vi "Automatic CE-CERT Inverter MODBUS TCP-IP Curtailment and Power Factor (Reduced Time)v2(multiple inverters).vi"() -> ()   [LabVIEW 2018]
uses:
  7c97fb1c-71e2-46b6-83e0-b90824be2fa8.vi
  af948a96-4452-4f5d-91ce-aeaf404a94af.vi
  83a0a89a-57e4-4031-9348-eb6639a1bf24.vi
  f3cab8c3-2d05-4b9a-baf3-8a451c362fa6.vi
  3941be6d-a080-493a-893c-1af352c84378.vi
  1a821f27-6730-4aaa-ab64-43c28f9c5f35.vi
  749368e9-8a13-4457-ac74-086f0bb157c2.vi
  1ca09a49-d2c4-4d2a-8422-a7731fce5b7b.vi
  a7e399ce-82dc-48aa-a6e2-ac362b8dfa23.vi
  75f83434-2c83-437c-aa7d-48cbf84b3d36.vi
  6cf8bfcf-bab5-4fe0-9dd9-fe191ab04daa.vi
  010fc5d1-faf8-4fdd-ade0-65e49e8fa1d8.vi
  614cc60f-aada-4277-8735-aed6e9796954.vi
  2032eeee-5097-44a1-b1ee-3eaf9e39defa.vi
  4bf1f800-a3f2-4091-8e61-355c803042a3.vi
  9cb70969-7b0c-4217-9893-0bce95bddca2.vi
  a7de19d3-9b8c-4fa7-88a3-467bd0df0b9d.vi
  8c202147-daa6-4192-8d63-29ec7b4b5446.vi
  <vilib>/Plasmionique/MB Master/MB_Master_TCP/MB_Master_TCP.lvclass
  C:/Program Files (x86)/National Instruments/LabVIEW 2018/vi.lib/Plasmionique/MB Master/MB_Master/MB_Master.lvclass
  <vilib>/Plasmionique/MB Master/MB Master.lvlib
panel:
  in  "1086 Inverter IP":string
  in  "1200 Inverter IP":string
  in  "Inverter Select":T1(ring)
  out "Setup Complete":bool
  in  "1084 Inverter IP":string
  out "Setup Runtime (s)":u32
  in  "Setup Curtailment and Power Factor":bool
  out "Curtailment Complete":bool
  out "Power Factor Complete":bool
  out "Power Factor Runtime (s)":u32
  out "Curtailment Runtime (s)":u32
  in  "Stop Button":bool
  in  "Send Power Factor":bool
  in  "Send Curtailment":bool
  in  "Curtailment % (28-100)":u16
  in  "Power Factor Setpoint":i32
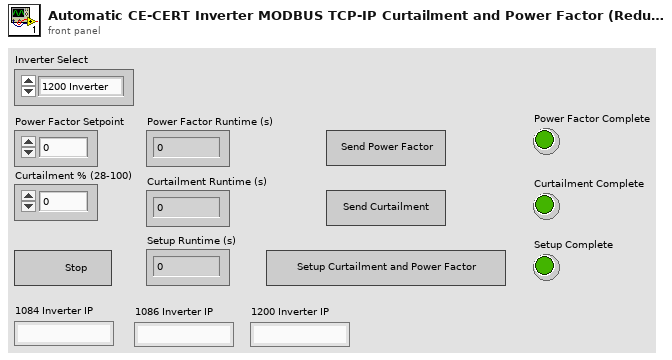
[diagram p1: front panel]
types:
  T1 = enum16{"1200 Inverter", "1084 Inverter", "1086 Inverter"}
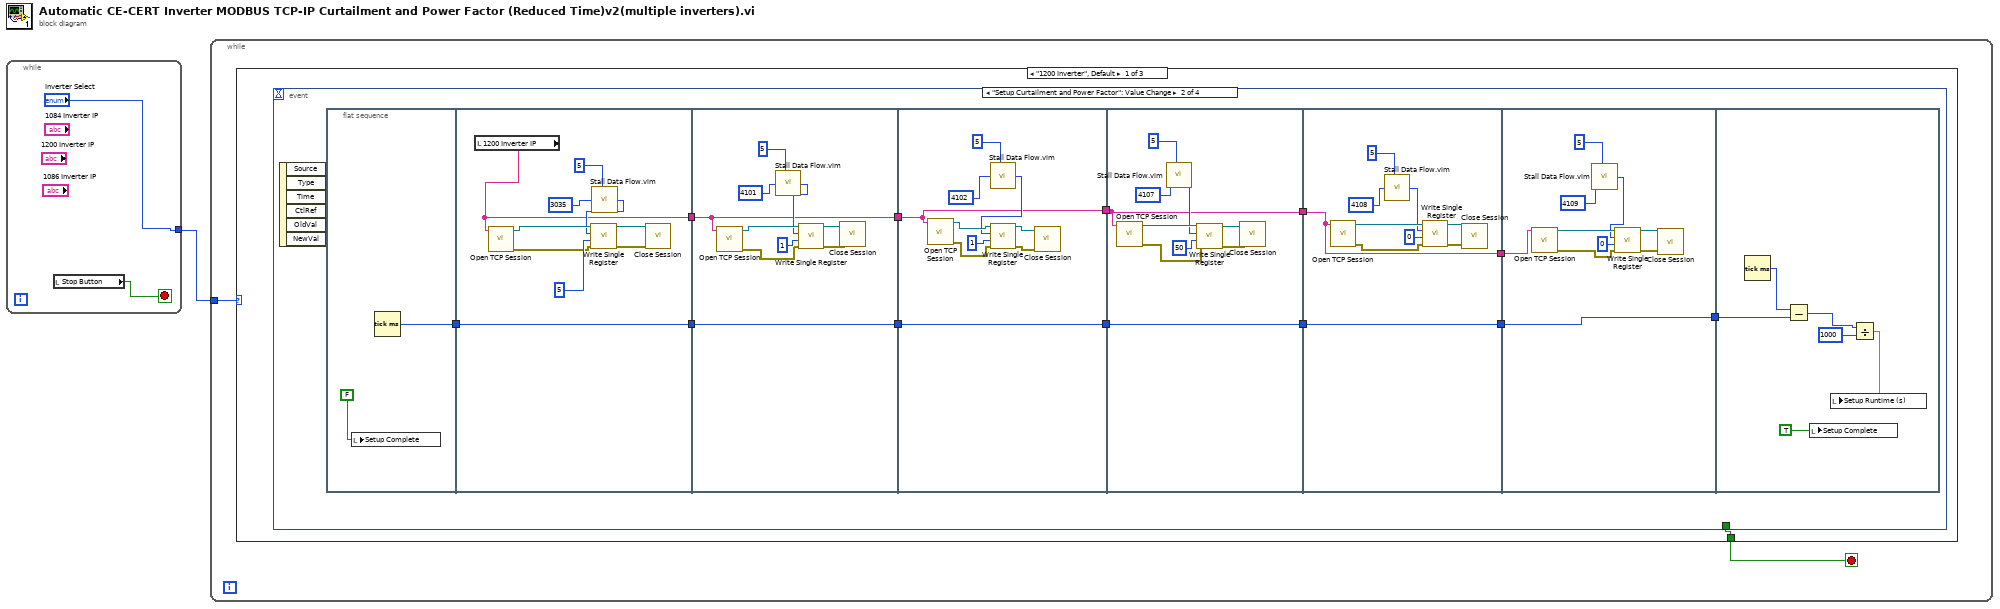
[diagram p0: block diagram]
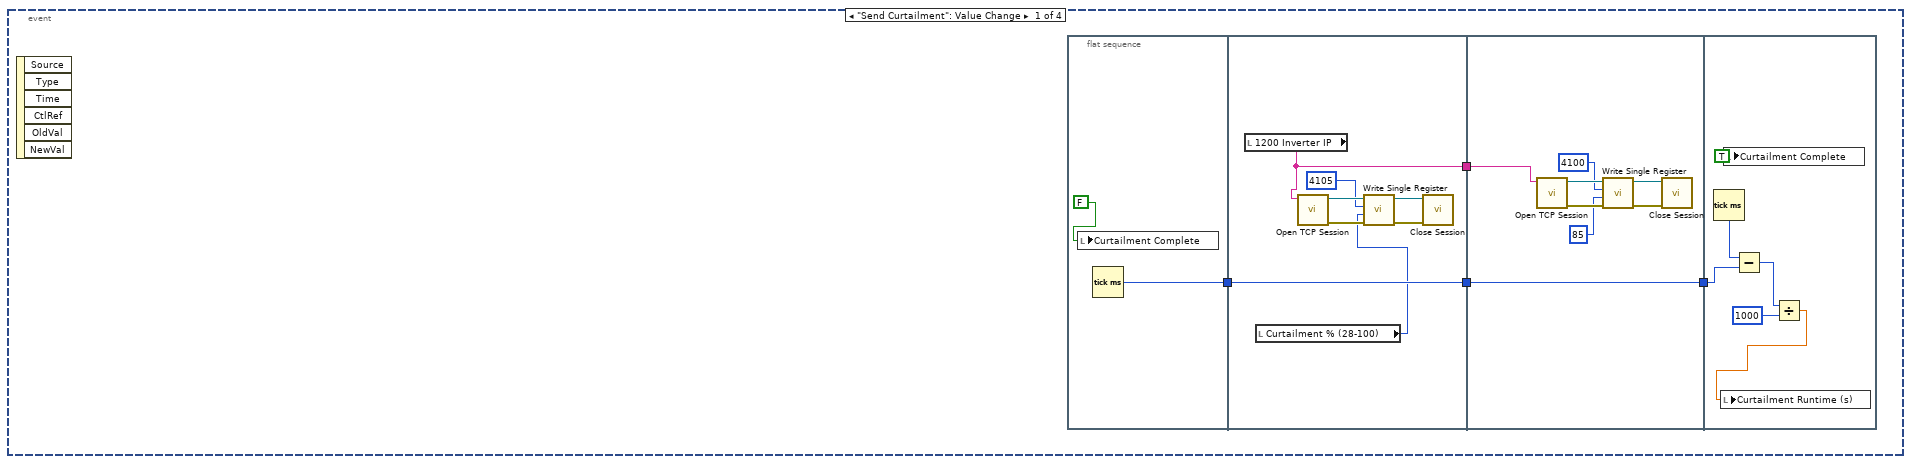
[diagram p2: hidden frame]
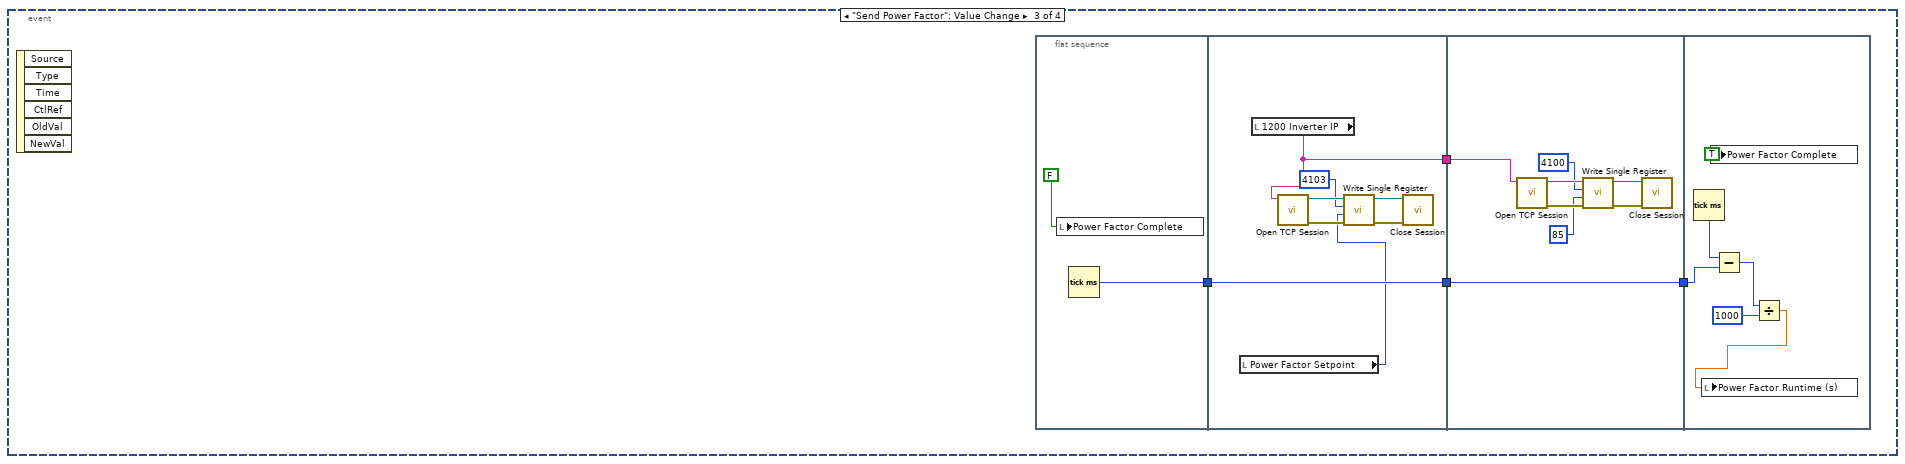
[diagram p3: hidden frame]
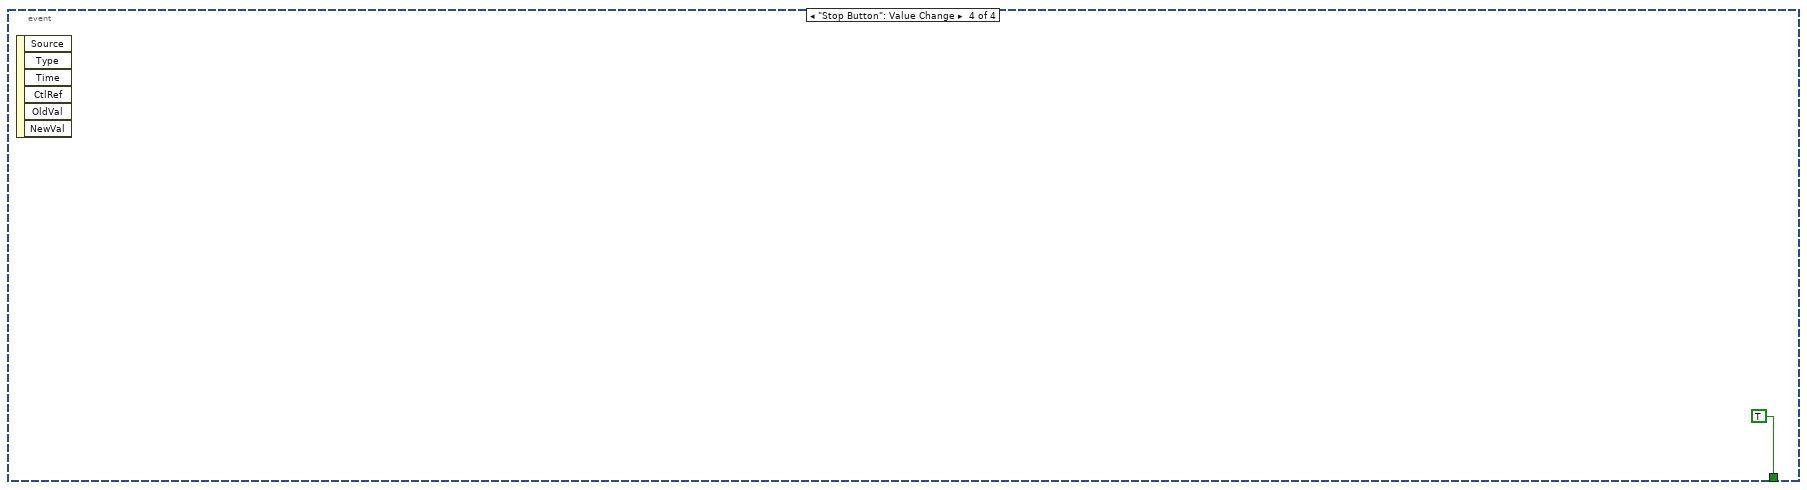
[diagram p4: hidden frame]
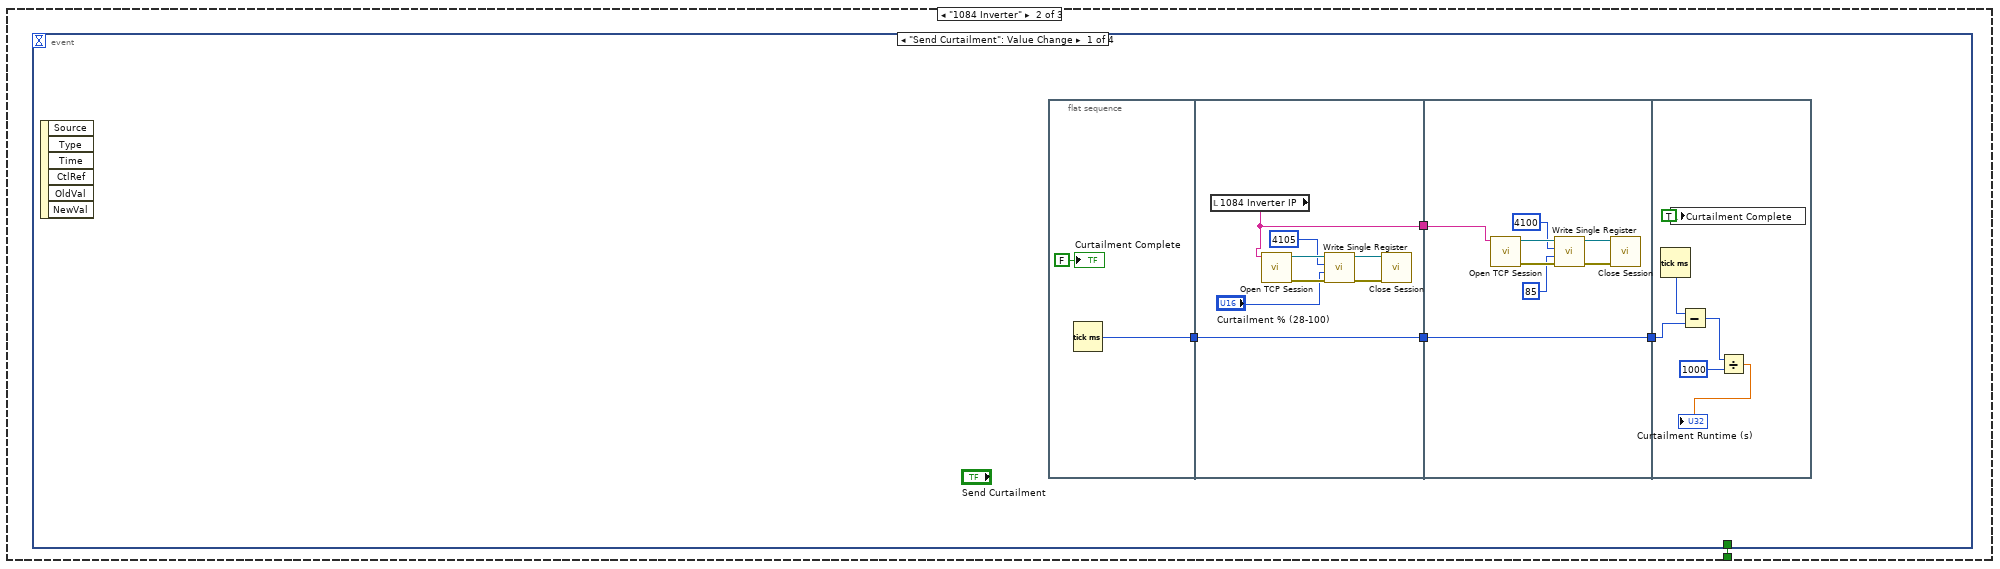
[diagram p5: hidden frame]
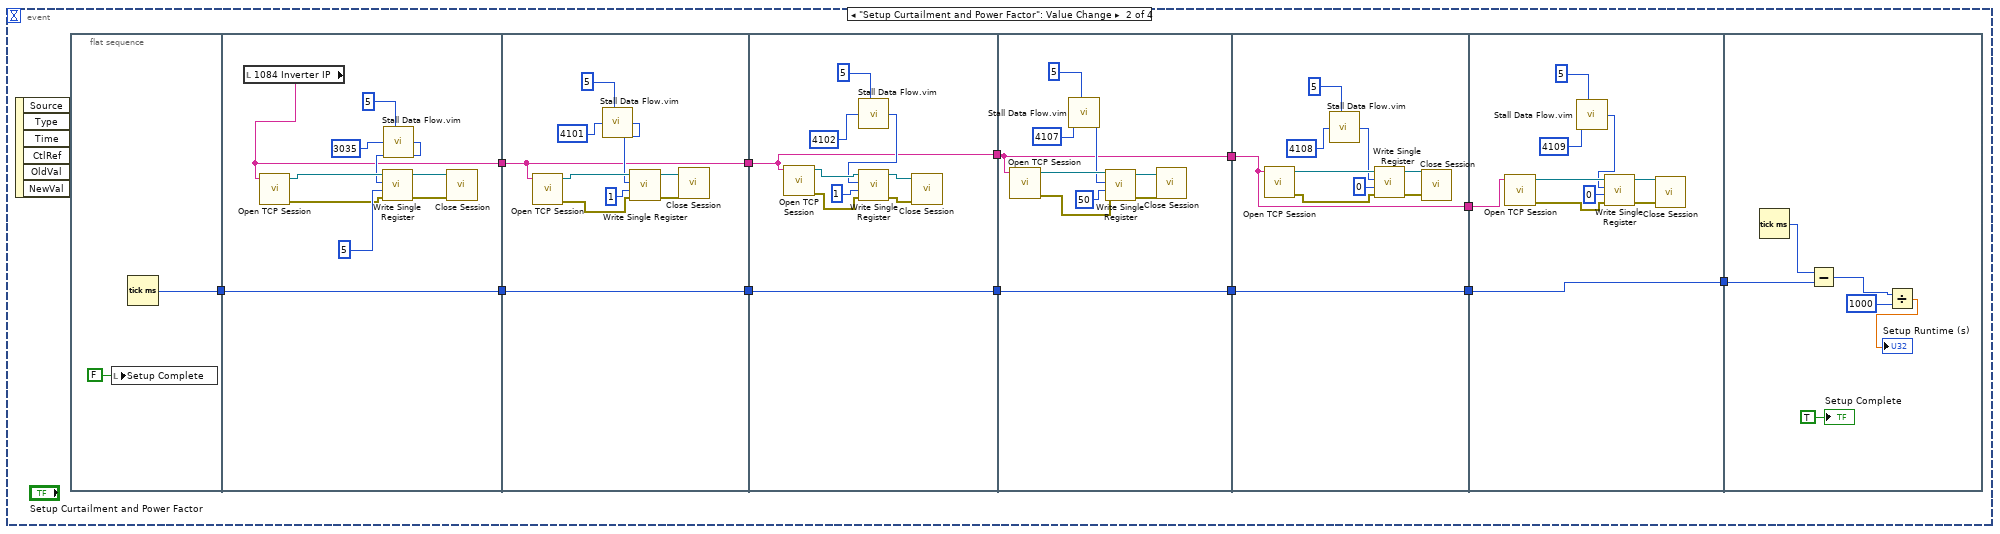
[diagram p6: hidden frame]
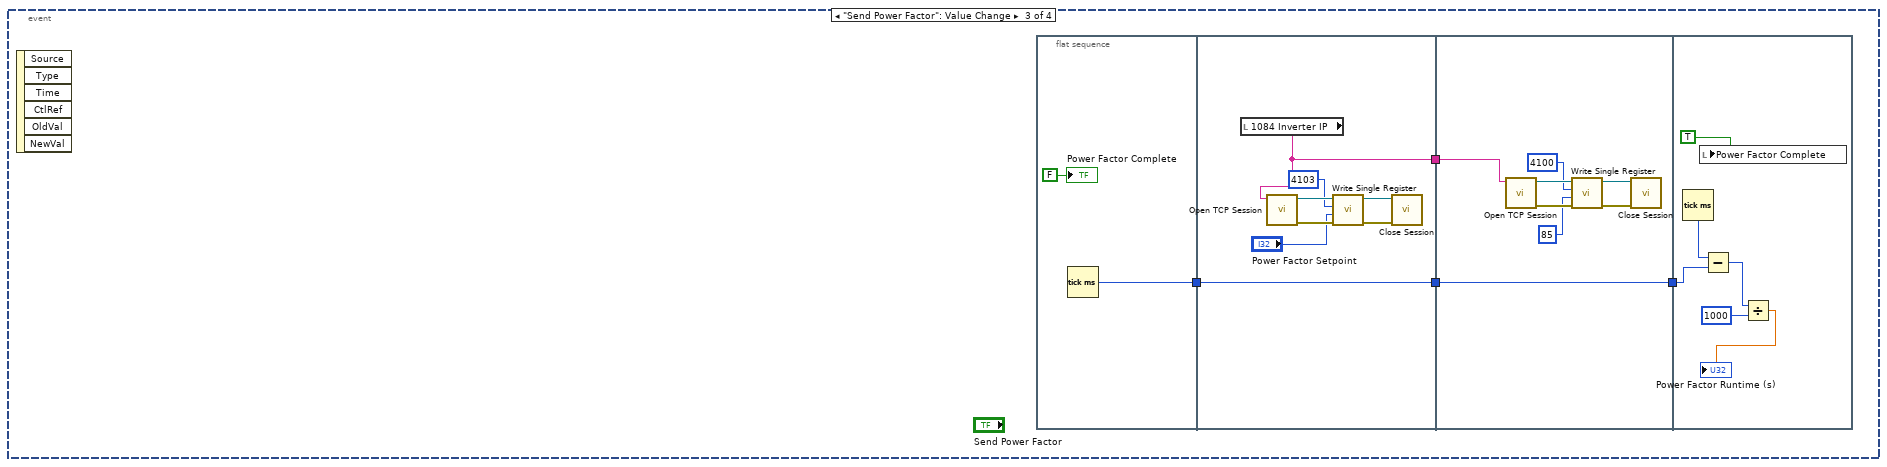
[diagram p7: hidden frame]
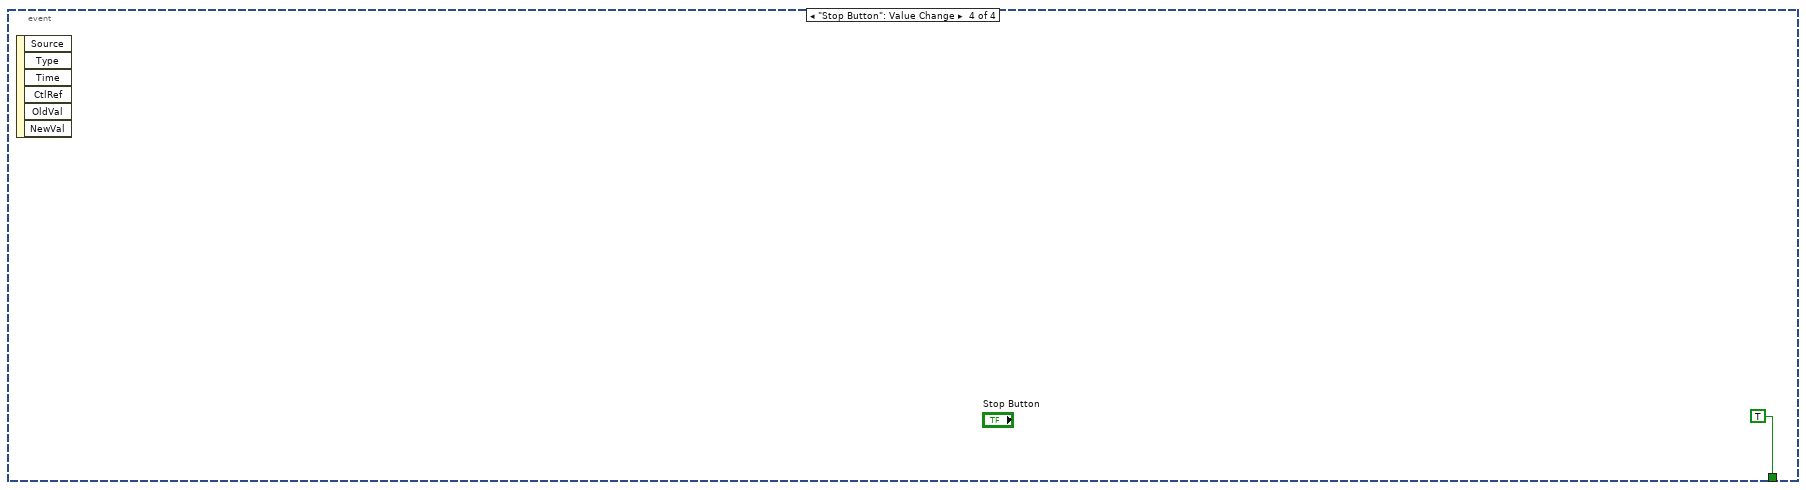
[diagram p8: hidden frame]
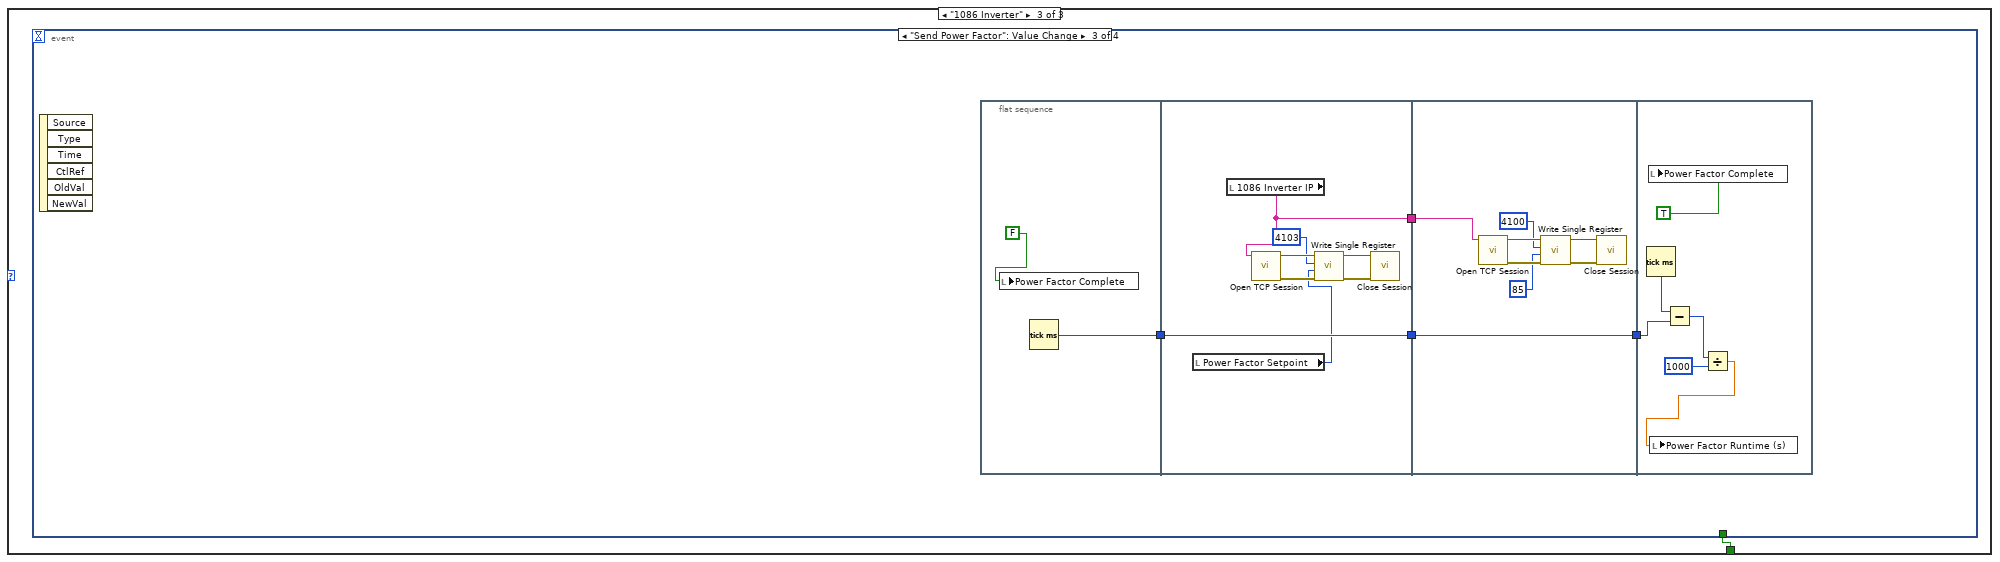
[diagram p9: hidden frame]
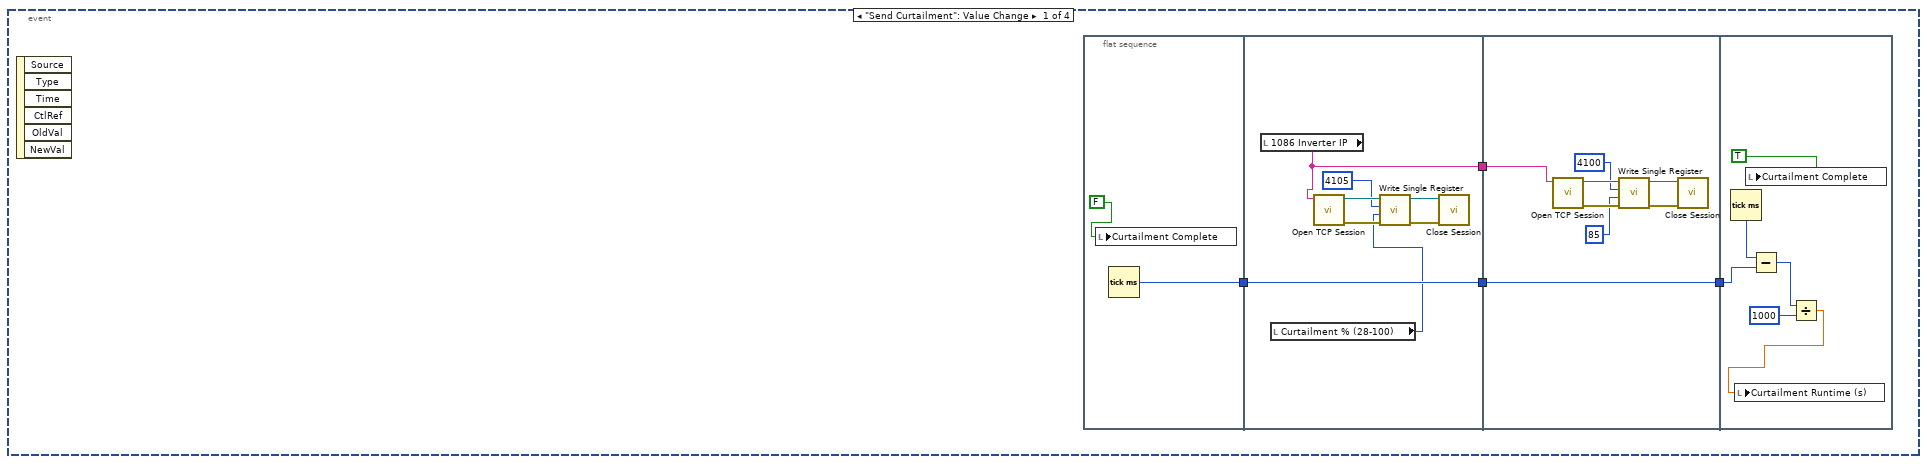
[diagram p10: hidden frame]
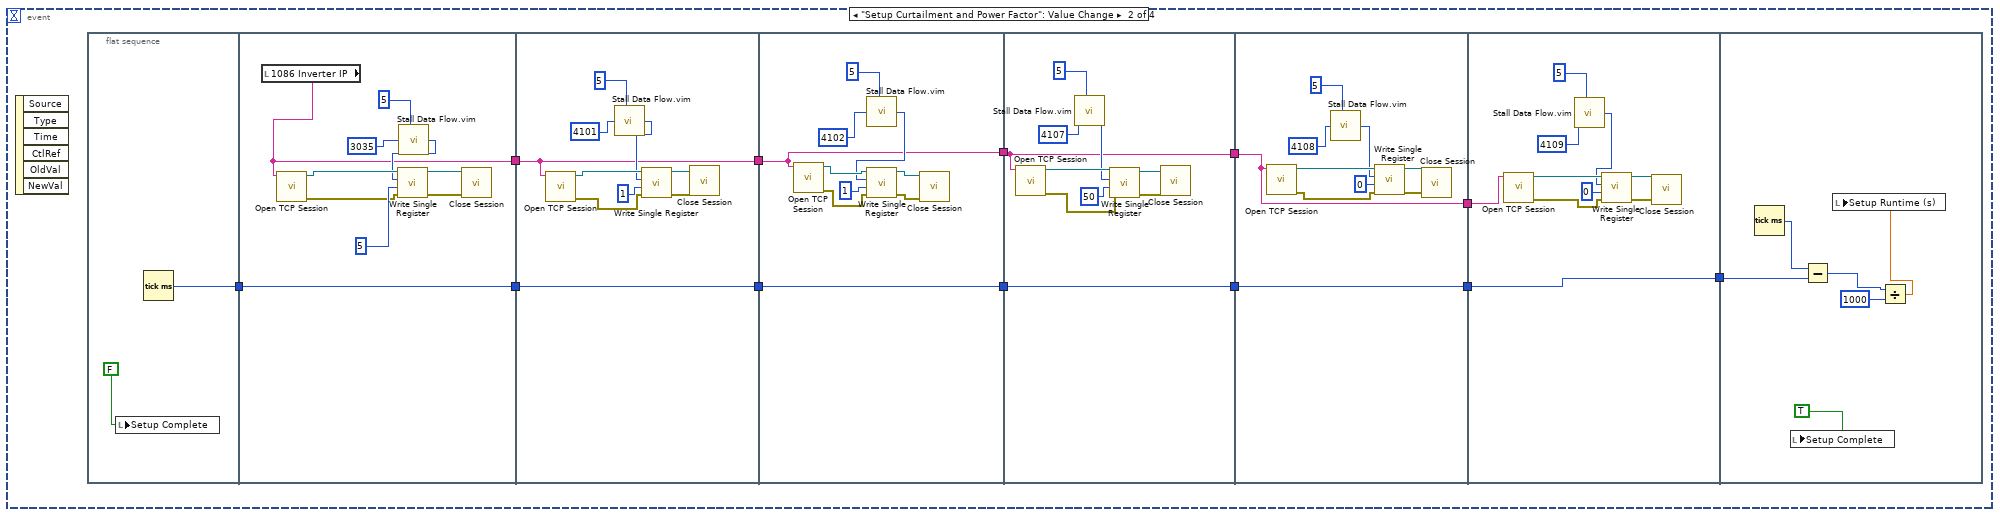
[diagram p11: hidden frame]
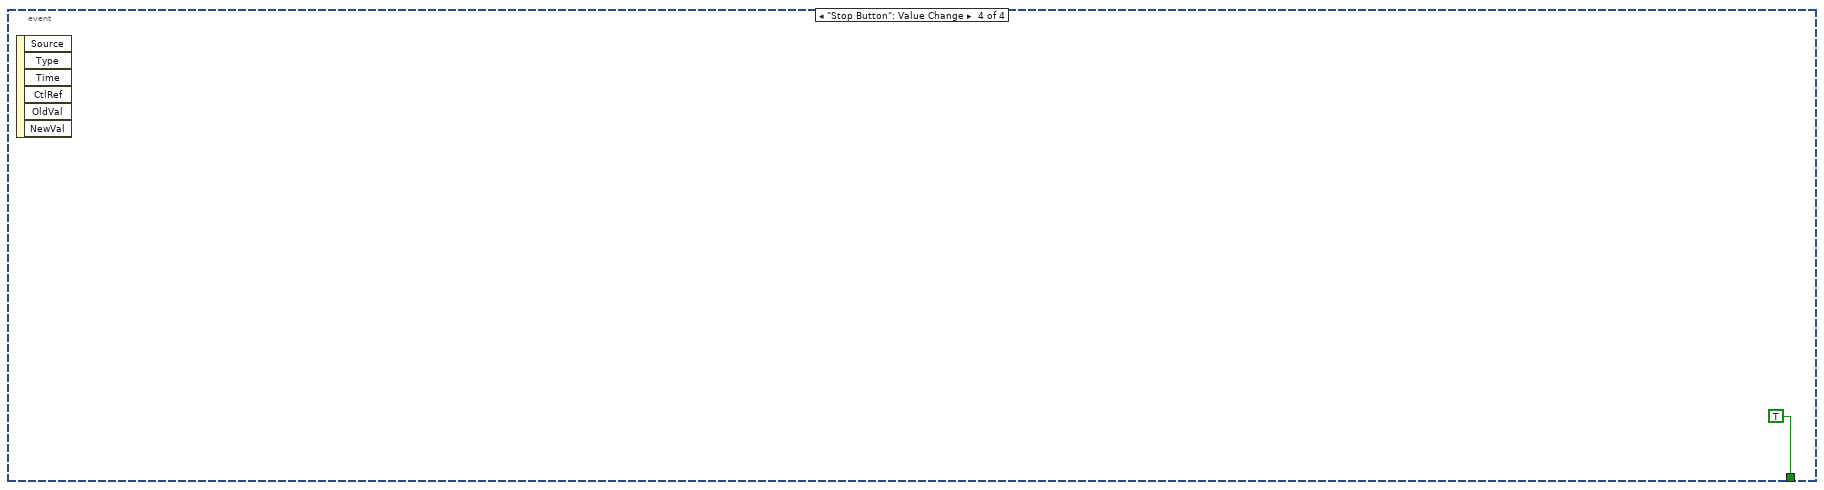
[diagram p12: hidden frame]
diagram:
  n1 = while {
    tunnel: ["Inverter Select"] -> w1
    stop <- w3 stop-if-true
    n2 = local read "Stop Button"() -> (w3:bool)
  }
  n3 = while {
    tunnel: w1 -> [w4]
    stop <- w5 stop-if-true
    n4 = case shown="\"1200 Inverter\", Default" w4 {
      tunnel: [w6 w144 w282] -> w5
      frame "1200 Inverter", Default {
        n5 = event shown="[1] \"Setup Curtailment and Power Factor\": Value Change" {
          selector: _ -> [_ _ _ _]
          dyn-events: _ -> [_ _ _ _]
          timeout: _ -> [_ _ _ _]
          tunnel: [_ _ _ TRUE] -> w6
          event "Send Curtailment": Value Change {
            n6 = event-data() -> ()  [unwired: 1 in, 6 out]
            n7 = flat-sequence {
              tunnel: [w12] -> w10
              tunnel: w10 -> [w15]
              tunnel: [w15] -> w8
              tunnel: [w14] -> w7
              tunnel: [w28] -> w9
              tunnel: w8 -> [w28]
              tunnel: w7 -> [w21]
              tunnel: w9 -> [w33]
              frame #0 {
                n8 = local write "Curtailment Complete"(FALSE ("Curtailment Sent")) -> ()
                n9 = Tick Count (ms)() -> (millisecond timer value=w12:u32)
              }
              frame #1 {
                n10 = local read "1200 Inverter IP"() -> (w14:string)
                n11 = local read "Curtailment % (28-100)"() -> (w13:u16)
                n12 = call <vilib>:"Open TCP Session.vi"("IP Address"=w14) -> ("error out"=w18:errorcluster, "MB_TCP session"=w20:refnum<class "MB_Master_TCP.lvclass">)  [unwired: 9 in]
                n13 = call <vilib>:"Write Single Register.vi"("error in (no error)"=w18, "value"=w13, "address"=u16 4105, "MB session in"=w20) -> ("error out"=w17:errorcluster, "MB session out"=w16:refnum<class "MB_Master_TCP.lvclass">)  [unwired: 6 in]
                n14 = call-dynamic "Close Session.vi"("error in (no error)"=w17, "MB TCP session"=w16) -> ()  [unwired: 9 in, 1 out]
              }
              frame #2 {
                n15 = call <vilib>:"Open TCP Session.vi"("IP Address"=w21) -> ("error out"=w25:errorcluster, "MB_TCP session"=w27:refnum<class "MB_Master_TCP.lvclass">)  [unwired: 9 in]
                n16 = call <vilib>:"Write Single Register.vi"("error in (no error)"=w25, "value"=u16 85, "address"=u16 4100, "MB session in"=w27) -> ("error out"=w24:errorcluster, "MB session out"=w23:refnum<class "MB_Master_TCP.lvclass">)  [unwired: 6 in]
                n17 = call-dynamic "Close Session.vi"("error in (no error)"=w24, "MB TCP session"=w23) -> ()  [unwired: 9 in, 1 out]
              }
              frame #3 {
                n18 = Tick Count (ms)() -> (millisecond timer value=w34:u32)
                n19 = local write "Curtailment Complete"(TRUE ("Curtailment Sent")) -> ()
                n20 = Subtract(x=w34, y=w33) -> (x-y=w32:u32)
                n21 = Divide(x=w32, y=u32 1000) -> (x/y=w29:dbl)
                n22 = local write "Curtailment Runtime (s)"(w29) -> ()
              }
            }
          }
          event "Setup Curtailment and Power Factor": Value Change {
            n23 = event-data() -> ()  [unwired: 1 in, 6 out]
            n24 = flat-sequence {
              tunnel: [w48] -> w46
              tunnel: [w50] -> w45
              tunnel: w46 -> [w50]
              tunnel: [w49] -> w44
              tunnel: [w60] -> w43
              tunnel: w45 -> [w60]
              tunnel: w44 -> [w59]
              tunnel: [w59] -> w42
              tunnel: [w70] -> w41
              tunnel: w43 -> [w70]
              tunnel: w42 -> [w69]
              tunnel: [w69] -> w40
              tunnel: [w80] -> w39
              tunnel: w41 -> [w80]
              tunnel: w40 -> [w79]
              tunnel: [w79] -> w38
              tunnel: [w90] -> w37
              tunnel: w39 -> [w90]
              tunnel: w38 -> [w89]
              tunnel: [w89] -> w36
              tunnel: w37 -> [w99]
              tunnel: w36 -> [w100]
              tunnel: [w99] -> w35
              tunnel: w35 -> [w113]
              frame #0 {
                n25 = local write "Setup Complete"(FALSE ("Setup Complete")) -> ()
                n26 = Tick Count (ms)() -> (millisecond timer value=w48:u32)
              }
              frame #1 {
                n27 = local read "1200 Inverter IP"() -> (w49:string)
                n28 = call <vilib>:"Open TCP Session.vi"("IP Address"=w49) -> ("error out"=w55:errorcluster, "MB_TCP session"=w54:refnum<class "MB_Master_TCP.lvclass">)  [unwired: 9 in]
                n29 = call "Stall Data Flow.vim"("value in"=u16 3035 ("address"), "milliseconds to wait"=u32 5) -> ("value out"=w51:u16)  [unwired: 1 out]
                n30 = call <vilib>:"Write Single Register.vi"("error in (no error)"=w55, "value"=u16 5, "address"=w51, "MB session in"=w54) -> ("error out"=w56:errorcluster, "MB session out"=w57:refnum<class "MB_Master_TCP.lvclass">)  [unwired: 6 in]
                n31 = call-dynamic "Close Session.vi"("error in (no error)"=w56, "MB TCP session"=w57) -> ()  [unwired: 9 in, 1 out]
              }
              frame #2 {
                n32 = call <vilib>:"Open TCP Session.vi"("IP Address"=w59) -> ("error out"=w66:errorcluster, "MB_TCP session"=w67:refnum<class "MB_Master_TCP.lvclass">)  [unwired: 9 in]
                n33 = call "Stall Data Flow.vim"("value in"=u16 4101 ("address"), "milliseconds to wait"=u32 5) -> ("value out"=w61:u16)  [unwired: 1 out]
                n34 = call <vilib>:"Write Single Register.vi"("error in (no error)"=w66, "value"=u16 1, "address"=w61, "MB session in"=w67) -> ("error out"=w65:errorcluster, "MB session out"=w64:refnum<class "MB_Master_TCP.lvclass">)  [unwired: 6 in]
                n35 = call-dynamic "Close Session.vi"("error in (no error)"=w65, "MB TCP session"=w64) -> ()  [unwired: 9 in, 1 out]
              }
              frame #3 {
                n36 = call <vilib>:"Open TCP Session.vi"("IP Address"=w69) -> ("error out"=w74:errorcluster, "MB_TCP session"=w77:refnum<class "MB_Master_TCP.lvclass">)  [unwired: 9 in]
                n37 = call "Stall Data Flow.vim"("value in"=u16 4102 ("address"), "milliseconds to wait"=u32 5) -> ("value out"=w71:u16)  [unwired: 1 out]
                n38 = call <vilib>:"Write Single Register.vi"("error in (no error)"=w74, "value"=u16 1, "address"=w71, "MB session in"=w77) -> ("error out"=w76:errorcluster, "MB session out"=w75:refnum<class "MB_Master_TCP.lvclass">)  [unwired: 6 in]
                n39 = call-dynamic "Close Session.vi"("error in (no error)"=w76, "MB TCP session"=w75) -> ()  [unwired: 9 in, 1 out]
              }
              frame #4 {
                n40 = call <vilib>:"Open TCP Session.vi"("IP Address"=w79) -> ("error out"=w84:errorcluster, "MB_TCP session"=w87:refnum<class "MB_Master_TCP.lvclass">)  [unwired: 9 in]
                n41 = call "Stall Data Flow.vim"("value in"=u16 4107 ("address"), "milliseconds to wait"=u32 5) -> ("value out"=w81:u16)  [unwired: 1 out]
                n42 = call <vilib>:"Write Single Register.vi"("error in (no error)"=w84, "value"=u16 50, "address"=w81, "MB session in"=w87) -> ("error out"=w86:errorcluster, "MB session out"=w85:refnum<class "MB_Master_TCP.lvclass">)  [unwired: 6 in]
                n43 = call-dynamic "Close Session.vi"("error in (no error)"=w86, "MB TCP session"=w85) -> ()  [unwired: 9 in, 1 out]
              }
              frame #5 {
                n44 = call <vilib>:"Open TCP Session.vi"("IP Address"=w89) -> ("error out"=w94:errorcluster, "MB_TCP session"=w97:refnum<class "MB_Master_TCP.lvclass">)  [unwired: 9 in]
                n45 = call "Stall Data Flow.vim"("value in"=u16 4108 ("address"), "milliseconds to wait"=u32 5) -> ("value out"=w92:u16)  [unwired: 1 out]
                n46 = call <vilib>:"Write Single Register.vi"("error in (no error)"=w94, "value"=u16 0, "address"=w92, "MB session in"=w97) -> ("error out"=w96:errorcluster, "MB session out"=w95:refnum<class "MB_Master_TCP.lvclass">)  [unwired: 6 in]
                n47 = call-dynamic "Close Session.vi"("error in (no error)"=w96, "MB TCP session"=w95) -> ()  [unwired: 9 in, 1 out]
              }
              frame #6 {
                n48 = call <vilib>:"Open TCP Session.vi"("IP Address"=w100) -> ("error out"=w106:errorcluster, "MB_TCP session"=w107:refnum<class "MB_Master_TCP.lvclass">)  [unwired: 9 in]
                n49 = call "Stall Data Flow.vim"("value in"=u16 4109 ("address"), "milliseconds to wait"=u32 5) -> ("value out"=w101:u16)  [unwired: 1 out]
                n50 = call <vilib>:"Write Single Register.vi"("error in (no error)"=w106, "value"=u16 0, "address"=w101, "MB session in"=w107) -> ("error out"=w104:errorcluster, "MB session out"=w105:refnum<class "MB_Master_TCP.lvclass">)  [unwired: 6 in]
                n51 = call-dynamic "Close Session.vi"("error in (no error)"=w104, "MB TCP session"=w105) -> ()  [unwired: 9 in, 1 out]
              }
              frame #7 {
                n52 = Tick Count (ms)() -> (millisecond timer value=w114:u32)
                n53 = Subtract(x=w114, y=w113) -> (x-y=w112:u32)
                n54 = local write "Setup Complete"(TRUE ("Setup Complete")) -> ()
                n55 = Divide(x=w112, y=u32 1000) -> (x/y=w109:dbl)
                n56 = local write "Setup Runtime (s)"(w109) -> ()
              }
            }
          }
          event "Send Power Factor": Value Change {
            n57 = event-data() -> ()  [unwired: 1 in, 6 out]
            n58 = flat-sequence {
              tunnel: [w120] -> w118
              tunnel: w118 -> [w123]
              tunnel: [w123] -> w117
              tunnel: [w122] -> w115
              tunnel: [w136] -> w116
              tunnel: w117 -> [w136]
              tunnel: w115 -> [w129]
              tunnel: w116 -> [w141]
              frame #0 {
                n59 = local write "Power Factor Complete"(FALSE ("Curtailment Sent")) -> ()
                n60 = Tick Count (ms)() -> (millisecond timer value=w120:u32)
              }
              frame #1 {
                n61 = local read "Power Factor Setpoint"() -> (w121:i32)
                n62 = local read "1200 Inverter IP"() -> (w122:string)
                n63 = call <vilib>:"Open TCP Session.vi"("IP Address"=w122) -> ("error out"=w126:errorcluster, "MB_TCP session"=w128:refnum<class "MB_Master_TCP.lvclass">)  [unwired: 9 in]
                n64 = call <vilib>:"Write Single Register.vi"("error in (no error)"=w126, "value"=w121, "address"=u16 4103, "MB session in"=w128) -> ("error out"=w125:errorcluster, "MB session out"=w124:refnum<class "MB_Master_TCP.lvclass">)  [unwired: 6 in]
                n65 = call-dynamic "Close Session.vi"("error in (no error)"=w125, "MB TCP session"=w124) -> ()  [unwired: 9 in, 1 out]
              }
              frame #2 {
                n66 = call <vilib>:"Open TCP Session.vi"("IP Address"=w129) -> ("error out"=w133:errorcluster, "MB_TCP session"=w135:refnum<class "MB_Master_TCP.lvclass">)  [unwired: 9 in]
                n67 = call <vilib>:"Write Single Register.vi"("error in (no error)"=w133, "value"=u16 85, "address"=u16 4100, "MB session in"=w135) -> ("error out"=w132:errorcluster, "MB session out"=w131:refnum<class "MB_Master_TCP.lvclass">)  [unwired: 6 in]
                n68 = call-dynamic "Close Session.vi"("error in (no error)"=w132, "MB TCP session"=w131) -> ()  [unwired: 9 in, 1 out]
              }
              frame #3 {
                n69 = Tick Count (ms)() -> (millisecond timer value=w142:u32)
                n70 = local write "Power Factor Complete"(TRUE ("Curtailment Sent")) -> ()
                n71 = Subtract(x=w142, y=w141) -> (x-y=w140:u32)
                n72 = Divide(x=w140, y=u32 1000) -> (x/y=w137:dbl)
                n73 = local write "Power Factor Runtime (s)"(w137) -> ()
              }
            }
          }
          event "Stop Button": Value Change {
            n74 = event-data() -> ()  [unwired: 1 in, 6 out]
          }
        }
      }
      frame "1084 Inverter" {
        n75 = event shown="[0] \"Send Curtailment\": Value Change" {
          selector: _ -> [_ _ _ _]
          dyn-events: _ -> [_ _ _ _]
          timeout: _ -> [_ _ _ _]
          tunnel: [_ _ _ TRUE] -> w144
          event "Send Curtailment": Value Change {
            n76 = event-data() -> ()  [unwired: 1 in, 6 out]
            n77 = flat-sequence {
              tunnel: [w150] -> w148
              tunnel: w148 -> [w153]
              tunnel: [w153] -> w146
              tunnel: [w151] -> w145
              tunnel: [w166] -> w147
              tunnel: w146 -> [w166]
              tunnel: w145 -> [w159]
              tunnel: w147 -> [w171]
              frame #0 {
                n78 = Tick Count (ms)() -> (millisecond timer value=w150:u32)
                "Curtailment Complete" <- FALSE ("Curtailment Sent")
              }
              frame #1 {
                n79 = local read "1084 Inverter IP"() -> (w151:string)
                n80 = call <vilib>:"Open TCP Session.vi"("IP Address"=w151) -> ("error out"=w156:errorcluster, "MB_TCP session"=w158:refnum<class "MB_Master_TCP.lvclass">)  [unwired: 9 in]
                n81 = call <vilib>:"Write Single Register.vi"("error in (no error)"=w156, "value"="Curtailment % (28-100)", "address"=u16 4105, "MB session in"=w158) -> ("error out"=w155:errorcluster, "MB session out"=w154:refnum<class "MB_Master_TCP.lvclass">)  [unwired: 6 in]
                n82 = call-dynamic "Close Session.vi"("error in (no error)"=w155, "MB TCP session"=w154) -> ()  [unwired: 9 in, 1 out]
              }
              frame #2 {
                n83 = call <vilib>:"Open TCP Session.vi"("IP Address"=w159) -> ("error out"=w163:errorcluster, "MB_TCP session"=w165:refnum<class "MB_Master_TCP.lvclass">)  [unwired: 9 in]
                n84 = call <vilib>:"Write Single Register.vi"("error in (no error)"=w163, "value"=u16 85, "address"=u16 4100, "MB session in"=w165) -> ("error out"=w162:errorcluster, "MB session out"=w161:refnum<class "MB_Master_TCP.lvclass">)  [unwired: 6 in]
                n85 = call-dynamic "Close Session.vi"("error in (no error)"=w162, "MB TCP session"=w161) -> ()  [unwired: 9 in, 1 out]
              }
              frame #3 {
                n86 = Tick Count (ms)() -> (millisecond timer value=w172:u32)
                n87 = local write "Curtailment Complete"(TRUE ("Curtailment Sent")) -> ()
                n88 = Subtract(x=w172, y=w171) -> (x-y=w170:u32)
                n89 = Divide(x=w170, y=u32 1000) -> (x/y=→"Curtailment Runtime (s)":dbl)
              }
            }
          }
          event "Setup Curtailment and Power Factor": Value Change {
            n90 = event-data() -> ()  [unwired: 1 in, 6 out]
            n91 = flat-sequence {
              tunnel: [w186] -> w184
              tunnel: [w188] -> w183
              tunnel: w184 -> [w188]
              tunnel: [w187] -> w182
              tunnel: [w198] -> w181
              tunnel: w183 -> [w198]
              tunnel: w182 -> [w197]
              tunnel: [w197] -> w180
              tunnel: [w208] -> w179
              tunnel: w181 -> [w208]
              tunnel: w180 -> [w207]
              tunnel: [w207] -> w178
              tunnel: [w218] -> w177
              tunnel: w179 -> [w218]
              tunnel: w178 -> [w217]
              tunnel: [w217] -> w176
              tunnel: [w228] -> w175
              tunnel: w177 -> [w228]
              tunnel: w176 -> [w227]
              tunnel: [w227] -> w174
              tunnel: w175 -> [w237]
              tunnel: w174 -> [w238]
              tunnel: [w237] -> w173
              tunnel: w173 -> [w251]
              frame #0 {
                n92 = local write "Setup Complete"(FALSE ("Setup Complete")) -> ()
                n93 = Tick Count (ms)() -> (millisecond timer value=w186:u32)
              }
              frame #1 {
                n94 = local read "1084 Inverter IP"() -> (w187:string)
                n95 = call <vilib>:"Open TCP Session.vi"("IP Address"=w187) -> ("error out"=w193:errorcluster, "MB_TCP session"=w192:refnum<class "MB_Master_TCP.lvclass">)  [unwired: 9 in]
                n96 = call "Stall Data Flow.vim"("value in"=u16 3035 ("address"), "milliseconds to wait"=u32 5) -> ("value out"=w189:u16)  [unwired: 1 out]
                n97 = call <vilib>:"Write Single Register.vi"("error in (no error)"=w193, "value"=u16 5, "address"=w189, "MB session in"=w192) -> ("error out"=w194:errorcluster, "MB session out"=w195:refnum<class "MB_Master_TCP.lvclass">)  [unwired: 6 in]
                n98 = call-dynamic "Close Session.vi"("error in (no error)"=w194, "MB TCP session"=w195) -> ()  [unwired: 9 in, 1 out]
              }
              frame #2 {
                n99 = call <vilib>:"Open TCP Session.vi"("IP Address"=w197) -> ("error out"=w204:errorcluster, "MB_TCP session"=w205:refnum<class "MB_Master_TCP.lvclass">)  [unwired: 9 in]
                n100 = call "Stall Data Flow.vim"("value in"=u16 4101 ("address"), "milliseconds to wait"=u32 5) -> ("value out"=w199:u16)  [unwired: 1 out]
                n101 = call <vilib>:"Write Single Register.vi"("error in (no error)"=w204, "value"=u16 1, "address"=w199, "MB session in"=w205) -> ("error out"=w203:errorcluster, "MB session out"=w202:refnum<class "MB_Master_TCP.lvclass">)  [unwired: 6 in]
                n102 = call-dynamic "Close Session.vi"("error in (no error)"=w203, "MB TCP session"=w202) -> ()  [unwired: 9 in, 1 out]
              }
              frame #3 {
                n103 = call <vilib>:"Open TCP Session.vi"("IP Address"=w207) -> ("error out"=w212:errorcluster, "MB_TCP session"=w215:refnum<class "MB_Master_TCP.lvclass">)  [unwired: 9 in]
                n104 = call "Stall Data Flow.vim"("value in"=u16 4102 ("address"), "milliseconds to wait"=u32 5) -> ("value out"=w209:u16)  [unwired: 1 out]
                n105 = call <vilib>:"Write Single Register.vi"("error in (no error)"=w212, "value"=u16 1, "address"=w209, "MB session in"=w215) -> ("error out"=w214:errorcluster, "MB session out"=w213:refnum<class "MB_Master_TCP.lvclass">)  [unwired: 6 in]
                n106 = call-dynamic "Close Session.vi"("error in (no error)"=w214, "MB TCP session"=w213) -> ()  [unwired: 9 in, 1 out]
              }
              frame #4 {
                n107 = call <vilib>:"Open TCP Session.vi"("IP Address"=w217) -> ("error out"=w222:errorcluster, "MB_TCP session"=w225:refnum<class "MB_Master_TCP.lvclass">)  [unwired: 9 in]
                n108 = call "Stall Data Flow.vim"("value in"=u16 4107 ("address"), "milliseconds to wait"=u32 5) -> ("value out"=w219:u16)  [unwired: 1 out]
                n109 = call <vilib>:"Write Single Register.vi"("error in (no error)"=w222, "value"=u16 50, "address"=w219, "MB session in"=w225) -> ("error out"=w224:errorcluster, "MB session out"=w223:refnum<class "MB_Master_TCP.lvclass">)  [unwired: 6 in]
                n110 = call-dynamic "Close Session.vi"("error in (no error)"=w224, "MB TCP session"=w223) -> ()  [unwired: 9 in, 1 out]
              }
              frame #5 {
                n111 = call <vilib>:"Open TCP Session.vi"("IP Address"=w227) -> ("error out"=w232:errorcluster, "MB_TCP session"=w235:refnum<class "MB_Master_TCP.lvclass">)  [unwired: 9 in]
                n112 = call "Stall Data Flow.vim"("value in"=u16 4108 ("address"), "milliseconds to wait"=u32 5) -> ("value out"=w230:u16)  [unwired: 1 out]
                n113 = call <vilib>:"Write Single Register.vi"("error in (no error)"=w232, "value"=u16 0, "address"=w230, "MB session in"=w235) -> ("error out"=w234:errorcluster, "MB session out"=w233:refnum<class "MB_Master_TCP.lvclass">)  [unwired: 6 in]
                n114 = call-dynamic "Close Session.vi"("error in (no error)"=w234, "MB TCP session"=w233) -> ()  [unwired: 9 in, 1 out]
              }
              frame #6 {
                n115 = call <vilib>:"Open TCP Session.vi"("IP Address"=w238) -> ("error out"=w244:errorcluster, "MB_TCP session"=w245:refnum<class "MB_Master_TCP.lvclass">)  [unwired: 9 in]
                n116 = call "Stall Data Flow.vim"("value in"=u16 4109 ("address"), "milliseconds to wait"=u32 5) -> ("value out"=w239:u16)  [unwired: 1 out]
                n117 = call <vilib>:"Write Single Register.vi"("error in (no error)"=w244, "value"=u16 0, "address"=w239, "MB session in"=w245) -> ("error out"=w242:errorcluster, "MB session out"=w243:refnum<class "MB_Master_TCP.lvclass">)  [unwired: 6 in]
                n118 = call-dynamic "Close Session.vi"("error in (no error)"=w242, "MB TCP session"=w243) -> ()  [unwired: 9 in, 1 out]
              }
              frame #7 {
                n119 = Tick Count (ms)() -> (millisecond timer value=w252:u32)
                n120 = Subtract(x=w252, y=w251) -> (x-y=w250:u32)
                n121 = Divide(x=w250, y=u32 1000) -> (x/y=→"Setup Runtime (s)":dbl)
                "Setup Complete" <- TRUE ("Setup Complete")
              }
            }
          }
          event "Send Power Factor": Value Change {
            n122 = event-data() -> ()  [unwired: 1 in, 6 out]
            n123 = flat-sequence {
              tunnel: [w258] -> w256
              tunnel: w256 -> [w261]
              tunnel: [w261] -> w255
              tunnel: [w259] -> w253
              tunnel: [w274] -> w254
              tunnel: w255 -> [w274]
              tunnel: w253 -> [w267]
              tunnel: w254 -> [w279]
              frame #0 {
                n124 = Tick Count (ms)() -> (millisecond timer value=w258:u32)
                "Power Factor Complete" <- FALSE ("Curtailment Sent")
              }
              frame #1 {
                n125 = local read "1084 Inverter IP"() -> (w259:string)
                n126 = call <vilib>:"Open TCP Session.vi"("IP Address"=w259) -> ("error out"=w264:errorcluster, "MB_TCP session"=w266:refnum<class "MB_Master_TCP.lvclass">)  [unwired: 9 in]
                n127 = call <vilib>:"Write Single Register.vi"("error in (no error)"=w264, "value"="Power Factor Setpoint", "address"=u16 4103, "MB session in"=w266) -> ("error out"=w263:errorcluster, "MB session out"=w262:refnum<class "MB_Master_TCP.lvclass">)  [unwired: 6 in]
                n128 = call-dynamic "Close Session.vi"("error in (no error)"=w263, "MB TCP session"=w262) -> ()  [unwired: 9 in, 1 out]
              }
              frame #2 {
                n129 = call <vilib>:"Open TCP Session.vi"("IP Address"=w267) -> ("error out"=w271:errorcluster, "MB_TCP session"=w273:refnum<class "MB_Master_TCP.lvclass">)  [unwired: 9 in]
                n130 = call <vilib>:"Write Single Register.vi"("error in (no error)"=w271, "value"=u16 85, "address"=u16 4100, "MB session in"=w273) -> ("error out"=w270:errorcluster, "MB session out"=w269:refnum<class "MB_Master_TCP.lvclass">)  [unwired: 6 in]
                n131 = call-dynamic "Close Session.vi"("error in (no error)"=w270, "MB TCP session"=w269) -> ()  [unwired: 9 in, 1 out]
              }
              frame #3 {
                n132 = Tick Count (ms)() -> (millisecond timer value=w280:u32)
                n133 = local write "Power Factor Complete"(TRUE ("Curtailment Sent")) -> ()
                n134 = Subtract(x=w280, y=w279) -> (x-y=w278:u32)
                n135 = Divide(x=w278, y=u32 1000) -> (x/y=→"Power Factor Runtime (s)":dbl)
              }
            }
          }
          event "Stop Button": Value Change {
            n136 = event-data() -> ()  [unwired: 1 in, 6 out]
          }
        }
      }
      frame "1086 Inverter" {
        n137 = event shown="[2] \"Send Power Factor\": Value Change" {
          selector: _ -> [_ _ _ _]
          dyn-events: _ -> [_ _ _ _]
          timeout: _ -> [_ _ _ _]
          tunnel: [_ _ _ TRUE] -> w282
          event "Send Curtailment": Value Change {
            n138 = event-data() -> ()  [unwired: 1 in, 6 out]
            n139 = flat-sequence {
              tunnel: [w288] -> w286
              tunnel: w286 -> [w291]
              tunnel: [w291] -> w284
              tunnel: [w290] -> w283
              tunnel: [w304] -> w285
              tunnel: w284 -> [w304]
              tunnel: w283 -> [w297]
              tunnel: w285 -> [w309]
              frame #0 {
                n140 = local write "Curtailment Complete"(FALSE ("Curtailment Sent")) -> ()
                n141 = Tick Count (ms)() -> (millisecond timer value=w288:u32)
              }
              frame #1 {
                n142 = local read "1086 Inverter IP"() -> (w290:string)
                n143 = local read "Curtailment % (28-100)"() -> (w289:u16)
                n144 = call <vilib>:"Open TCP Session.vi"("IP Address"=w290) -> ("error out"=w294:errorcluster, "MB_TCP session"=w296:refnum<class "MB_Master_TCP.lvclass">)  [unwired: 9 in]
                n145 = call <vilib>:"Write Single Register.vi"("error in (no error)"=w294, "value"=w289, "address"=u16 4105, "MB session in"=w296) -> ("error out"=w293:errorcluster, "MB session out"=w292:refnum<class "MB_Master_TCP.lvclass">)  [unwired: 6 in]
                n146 = call-dynamic "Close Session.vi"("error in (no error)"=w293, "MB TCP session"=w292) -> ()  [unwired: 9 in, 1 out]
              }
              frame #2 {
                n147 = call <vilib>:"Open TCP Session.vi"("IP Address"=w297) -> ("error out"=w301:errorcluster, "MB_TCP session"=w303:refnum<class "MB_Master_TCP.lvclass">)  [unwired: 9 in]
                n148 = call <vilib>:"Write Single Register.vi"("error in (no error)"=w301, "value"=u16 85, "address"=u16 4100, "MB session in"=w303) -> ("error out"=w300:errorcluster, "MB session out"=w299:refnum<class "MB_Master_TCP.lvclass">)  [unwired: 6 in]
                n149 = call-dynamic "Close Session.vi"("error in (no error)"=w300, "MB TCP session"=w299) -> ()  [unwired: 9 in, 1 out]
              }
              frame #3 {
                n150 = Tick Count (ms)() -> (millisecond timer value=w310:u32)
                n151 = local write "Curtailment Complete"(TRUE ("Curtailment Sent")) -> ()
                n152 = Subtract(x=w310, y=w309) -> (x-y=w308:u32)
                n153 = Divide(x=w308, y=u32 1000) -> (x/y=w305:dbl)
                n154 = local write "Curtailment Runtime (s)"(w305) -> ()
              }
            }
          }
          event "Setup Curtailment and Power Factor": Value Change {
            n155 = event-data() -> ()  [unwired: 1 in, 6 out]
            n156 = flat-sequence {
              tunnel: [w324] -> w322
              tunnel: [w326] -> w321
              tunnel: w322 -> [w326]
              tunnel: [w325] -> w320
              tunnel: [w336] -> w319
              tunnel: w321 -> [w336]
              tunnel: w320 -> [w335]
              tunnel: [w335] -> w318
              tunnel: [w346] -> w317
              tunnel: w319 -> [w346]
              tunnel: w318 -> [w345]
              tunnel: [w345] -> w316
              tunnel: [w356] -> w315
              tunnel: w317 -> [w356]
              tunnel: w316 -> [w355]
              tunnel: [w355] -> w314
              tunnel: [w366] -> w313
              tunnel: w315 -> [w366]
              tunnel: w314 -> [w365]
              tunnel: [w365] -> w312
              tunnel: w313 -> [w375]
              tunnel: w312 -> [w376]
              tunnel: [w375] -> w311
              tunnel: w311 -> [w389]
              frame #0 {
                n157 = local write "Setup Complete"(FALSE ("Setup Complete")) -> ()
                n158 = Tick Count (ms)() -> (millisecond timer value=w324:u32)
              }
              frame #1 {
                n159 = local read "1086 Inverter IP"() -> (w325:string)
                n160 = call <vilib>:"Open TCP Session.vi"("IP Address"=w325) -> ("error out"=w331:errorcluster, "MB_TCP session"=w330:refnum<class "MB_Master_TCP.lvclass">)  [unwired: 9 in]
                n161 = call "Stall Data Flow.vim"("value in"=u16 3035 ("address"), "milliseconds to wait"=u32 5) -> ("value out"=w327:u16)  [unwired: 1 out]
                n162 = call <vilib>:"Write Single Register.vi"("error in (no error)"=w331, "value"=u16 5, "address"=w327, "MB session in"=w330) -> ("error out"=w332:errorcluster, "MB session out"=w333:refnum<class "MB_Master_TCP.lvclass">)  [unwired: 6 in]
                n163 = call-dynamic "Close Session.vi"("error in (no error)"=w332, "MB TCP session"=w333) -> ()  [unwired: 9 in, 1 out]
              }
              frame #2 {
                n164 = call <vilib>:"Open TCP Session.vi"("IP Address"=w335) -> ("error out"=w342:errorcluster, "MB_TCP session"=w343:refnum<class "MB_Master_TCP.lvclass">)  [unwired: 9 in]
                n165 = call "Stall Data Flow.vim"("value in"=u16 4101 ("address"), "milliseconds to wait"=u32 5) -> ("value out"=w337:u16)  [unwired: 1 out]
                n166 = call <vilib>:"Write Single Register.vi"("error in (no error)"=w342, "value"=u16 1, "address"=w337, "MB session in"=w343) -> ("error out"=w341:errorcluster, "MB session out"=w340:refnum<class "MB_Master_TCP.lvclass">)  [unwired: 6 in]
                n167 = call-dynamic "Close Session.vi"("error in (no error)"=w341, "MB TCP session"=w340) -> ()  [unwired: 9 in, 1 out]
              }
              frame #3 {
                n168 = call <vilib>:"Open TCP Session.vi"("IP Address"=w345) -> ("error out"=w350:errorcluster, "MB_TCP session"=w353:refnum<class "MB_Master_TCP.lvclass">)  [unwired: 9 in]
                n169 = call "Stall Data Flow.vim"("value in"=u16 4102 ("address"), "milliseconds to wait"=u32 5) -> ("value out"=w347:u16)  [unwired: 1 out]
                n170 = call <vilib>:"Write Single Register.vi"("error in (no error)"=w350, "value"=u16 1, "address"=w347, "MB session in"=w353) -> ("error out"=w352:errorcluster, "MB session out"=w351:refnum<class "MB_Master_TCP.lvclass">)  [unwired: 6 in]
                n171 = call-dynamic "Close Session.vi"("error in (no error)"=w352, "MB TCP session"=w351) -> ()  [unwired: 9 in, 1 out]
              }
              frame #4 {
                n172 = call <vilib>:"Open TCP Session.vi"("IP Address"=w355) -> ("error out"=w360:errorcluster, "MB_TCP session"=w363:refnum<class "MB_Master_TCP.lvclass">)  [unwired: 9 in]
                n173 = call "Stall Data Flow.vim"("value in"=u16 4107 ("address"), "milliseconds to wait"=u32 5) -> ("value out"=w357:u16)  [unwired: 1 out]
                n174 = call <vilib>:"Write Single Register.vi"("error in (no error)"=w360, "value"=u16 50, "address"=w357, "MB session in"=w363) -> ("error out"=w362:errorcluster, "MB session out"=w361:refnum<class "MB_Master_TCP.lvclass">)  [unwired: 6 in]
                n175 = call-dynamic "Close Session.vi"("error in (no error)"=w362, "MB TCP session"=w361) -> ()  [unwired: 9 in, 1 out]
              }
              frame #5 {
                n176 = call <vilib>:"Open TCP Session.vi"("IP Address"=w365) -> ("error out"=w370:errorcluster, "MB_TCP session"=w373:refnum<class "MB_Master_TCP.lvclass">)  [unwired: 9 in]
                n177 = call "Stall Data Flow.vim"("value in"=u16 4108 ("address"), "milliseconds to wait"=u32 5) -> ("value out"=w368:u16)  [unwired: 1 out]
                n178 = call <vilib>:"Write Single Register.vi"("error in (no error)"=w370, "value"=u16 0, "address"=w368, "MB session in"=w373) -> ("error out"=w372:errorcluster, "MB session out"=w371:refnum<class "MB_Master_TCP.lvclass">)  [unwired: 6 in]
                n179 = call-dynamic "Close Session.vi"("error in (no error)"=w372, "MB TCP session"=w371) -> ()  [unwired: 9 in, 1 out]
              }
              frame #6 {
                n180 = call <vilib>:"Open TCP Session.vi"("IP Address"=w376) -> ("error out"=w382:errorcluster, "MB_TCP session"=w383:refnum<class "MB_Master_TCP.lvclass">)  [unwired: 9 in]
                n181 = call "Stall Data Flow.vim"("value in"=u16 4109 ("address"), "milliseconds to wait"=u32 5) -> ("value out"=w377:u16)  [unwired: 1 out]
                n182 = call <vilib>:"Write Single Register.vi"("error in (no error)"=w382, "value"=u16 0, "address"=w377, "MB session in"=w383) -> ("error out"=w380:errorcluster, "MB session out"=w381:refnum<class "MB_Master_TCP.lvclass">)  [unwired: 6 in]
                n183 = call-dynamic "Close Session.vi"("error in (no error)"=w380, "MB TCP session"=w381) -> ()  [unwired: 9 in, 1 out]
              }
              frame #7 {
                n184 = Tick Count (ms)() -> (millisecond timer value=w390:u32)
                n185 = local write "Setup Complete"(TRUE ("Setup Complete")) -> ()
                n186 = Subtract(x=w390, y=w389) -> (x-y=w388:u32)
                n187 = Divide(x=w388, y=u32 1000) -> (x/y=w386:dbl)
                n188 = local write "Setup Runtime (s)"(w386) -> ()
              }
            }
          }
          event "Send Power Factor": Value Change {
            n189 = event-data() -> ()  [unwired: 1 in, 6 out]
            n190 = flat-sequence {
              tunnel: [w396] -> w394
              tunnel: w394 -> [w399]
              tunnel: [w399] -> w393
              tunnel: [w398] -> w391
              tunnel: [w412] -> w392
              tunnel: w393 -> [w412]
              tunnel: w391 -> [w405]
              tunnel: w392 -> [w417]
              frame #0 {
                n191 = local write "Power Factor Complete"(FALSE ("Curtailment Sent")) -> ()
                n192 = Tick Count (ms)() -> (millisecond timer value=w396:u32)
              }
              frame #1 {
                n193 = local read "Power Factor Setpoint"() -> (w397:i32)
                n194 = local read "1086 Inverter IP"() -> (w398:string)
                n195 = call <vilib>:"Open TCP Session.vi"("IP Address"=w398) -> ("error out"=w402:errorcluster, "MB_TCP session"=w404:refnum<class "MB_Master_TCP.lvclass">)  [unwired: 9 in]
                n196 = call <vilib>:"Write Single Register.vi"("error in (no error)"=w402, "value"=w397, "address"=u16 4103, "MB session in"=w404) -> ("error out"=w401:errorcluster, "MB session out"=w400:refnum<class "MB_Master_TCP.lvclass">)  [unwired: 6 in]
                n197 = call-dynamic "Close Session.vi"("error in (no error)"=w401, "MB TCP session"=w400) -> ()  [unwired: 9 in, 1 out]
              }
              frame #2 {
                n198 = call <vilib>:"Open TCP Session.vi"("IP Address"=w405) -> ("error out"=w409:errorcluster, "MB_TCP session"=w411:refnum<class "MB_Master_TCP.lvclass">)  [unwired: 9 in]
                n199 = call <vilib>:"Write Single Register.vi"("error in (no error)"=w409, "value"=u16 85, "address"=u16 4100, "MB session in"=w411) -> ("error out"=w408:errorcluster, "MB session out"=w407:refnum<class "MB_Master_TCP.lvclass">)  [unwired: 6 in]
                n200 = call-dynamic "Close Session.vi"("error in (no error)"=w408, "MB TCP session"=w407) -> ()  [unwired: 9 in, 1 out]
              }
              frame #3 {
                n201 = Tick Count (ms)() -> (millisecond timer value=w418:u32)
                n202 = local write "Power Factor Complete"(TRUE ("Curtailment Sent")) -> ()
                n203 = Subtract(x=w418, y=w417) -> (x-y=w416:u32)
                n204 = Divide(x=w416, y=u32 1000) -> (x/y=w413:dbl)
                n205 = local write "Power Factor Runtime (s)"(w413) -> ()
              }
            }
          }
          event "Stop Button": Value Change {
            n206 = event-data() -> ()  [unwired: 1 in, 6 out]
          }
        }
      }
    }
  }
